vi "Initialize by XML.vi"(7 "XML File":path, 8 "error in (no error)":errorcluster, 10 "FPGA Device Address":string, 11 "FPGA Bitfile":path) -> (0 "error out":errorcluster, 3 "1553 Board out":refnum<class "1553 Board.lvclass">)   [LabVIEW 2016]
doc: "Generates a complete 1553 Board configuration when supplied a properly-formatted XML definition file.\n\nThe FPGA Bitfile must be one of the supported bitfiles that facilitates data communication with the 1553 Board. The FPGA Device Address must be a valid FPGA target."
uses:
  1553 Board.lvclass
  1553 Component/1553 Component.lvclass
  <vilib>/xml/NI_XML.lvlib
  <vilib>/xml/Load XML File.vi
  <vilib>/xml/Close Reference(Node).vi
  Utilities/FPGA Interface/FPGA Interface.lvclass
  Bus Controller/Bus Controller.lvclass
  D:/SVN/Products/BCI-1553/Software/Development/2016/Windows/1553 SubComponent/1553 SubComponent.lvclass
  Bus Monitor/Bus Monitor.lvclass
  Remote Terminal/Remote Terminal.lvclass
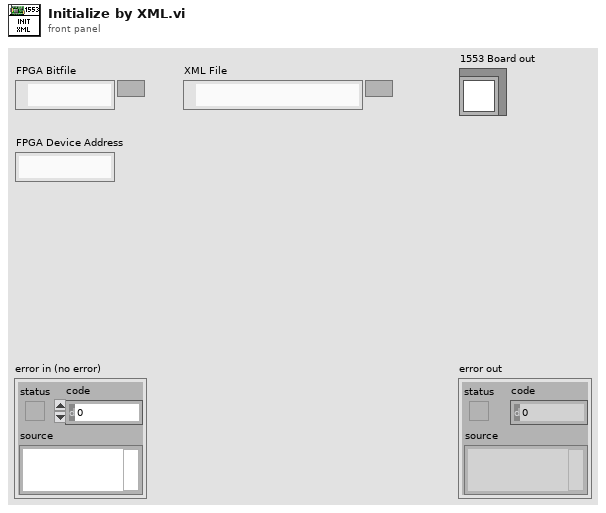
[diagram p1: front panel]
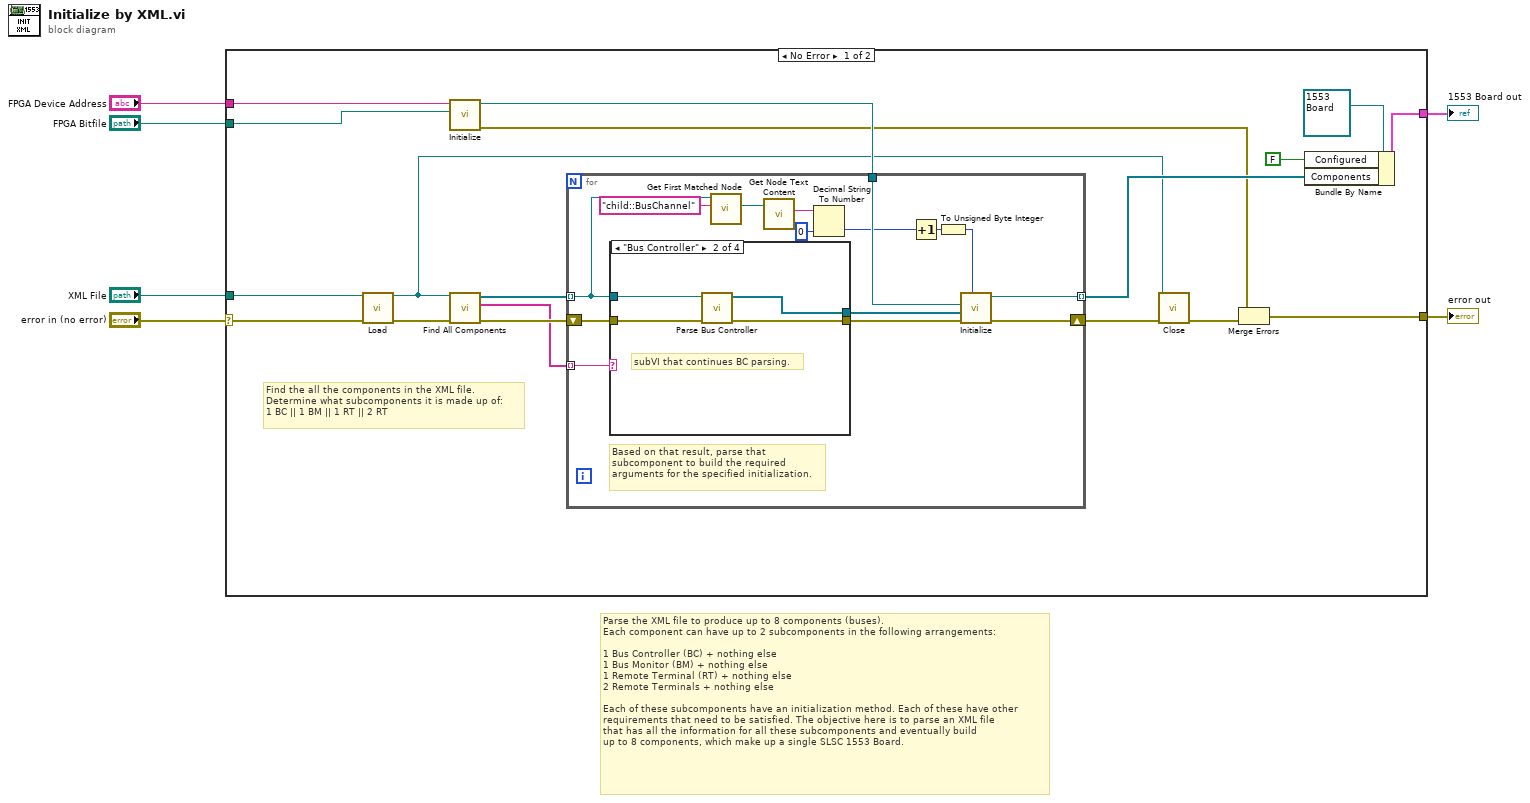
[diagram p0: block diagram]
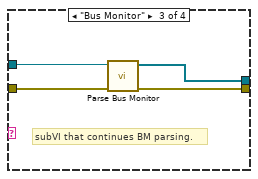
[diagram p3: hidden frame]
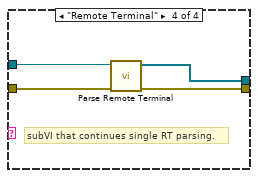
[diagram p4: hidden frame]
diagram:
  # "Parse the XML file to produce up to 8 components (buses).\nEach component can have up to 2 subcomponents in the following arrangements:\n\n1 Bus Controller (BC) + nothing else\n1 Bus Monitor (BM) + nothing else\n1 Remote Terminal (RT) + nothing else\n2 Remote Terminals + nothing else\n\nEach of these subcomponents have an initialization method. Each of these have other\nrequirements that need to be satisfied. The objective here is to parse an XML file\nthat has all the information for all these subcomponents and eventually build\nup to 8 components, which make up a single SLSC 1553 Board."
  n1 = case shown="No Error" "error in (no error)" {
    selector: "error in (no error)" -> [w16 w53]
    tunnel: [w7 w53] -> w5
    tunnel: [w23 _] -> w4
    tunnel: "FPGA Bitfile" -> [w21 _]
    tunnel: "FPGA Device Address" -> [w20 _]
    tunnel: "XML File" -> [w17 _]
    frame No Error {
      # "Find the all the components in the XML file.\nDetermine what subcomponents it is made up of:\n1 BC || 1 BM || 1 RT || 2 RT"
      n2 = call-poly <vilib>:"Load.vi"("path to XML document"=w17, "error in (no error)"=w16) -> ("DOM document out"=w14:refnum<k20>, "error out"=w13:errorcluster)  [unwired: 11 in, 1 out]
      n3 = call "Initialize.vi"("Bitfile path"=w21, "Device address"=w20) -> ("error out"=w9:errorcluster, "FPGA Interface out"=w19:refnum<class "FPGA Interface.lvclass">)  [unwired: 8 in]
      n4 = call "Find All Components.vi"("error in (no error)"=w13, "XML Doc Ref in"=w14) -> ("error out"=w12:errorcluster, "Component Types"=w10:string[], "Nodes"=w11:refnum<k20>[])  [unwired: 7 in]
      n5 = for {
        tunnel: w19 -> [w39]
        tunnel: [w31] -> w18 mode=indexing
        tunnel: w10 -> [w34] mode=indexing
        shift-right: [w38] -> w15
        shift-left: w12 -> [w33]
        tunnel: w11 -> [w30] mode=indexing
        # "Based on that result, parse that\nsubcomponent to build the required\narguments for the specified initialization."
        n6 = case shown="\"Bus Controller\"" w34 {
          tunnel: [w40 w42 w46 w50] -> w36
          tunnel: w33 -> [w40 w43 w48 w51]
          tunnel: [_ w41 w45 w49] -> w35
          tunnel: w30 -> [_ w44 w47 w52]
          frame Default {
            # "This case makes no sense.\nMake sure it doesn't get called."
          }
          frame "Bus Controller" {
            # "subVI that continues BC parsing."
            n7 = call "Parse Bus Controller.vi"("error in (no error)"=w43, "Bus Controller XML Node"=w44) -> ("error out"=w42:errorcluster, "Bus Controller"=w41:refnum<class "Bus Controller.lvclass">[])  [unwired: 8 in]
          }
          frame "Bus Monitor" {
            # "subVI that continues BM parsing."
            n8 = call "Parse Bus Monitor.vi"("error in (no error)"=w48, "Bus Monitor XML Node"=w47) -> ("error out"=w46:errorcluster, "Bus Monitor"=w45:refnum<class "Bus Monitor.lvclass">[])  [unwired: 8 in]
          }
          frame "Remote Terminal" {
            # "subVI that continues single RT parsing."
            n9 = call "Parse Remote Terminal.vi"("error in (no error)"=w51, "Single RT XML Node"=w52) -> ("error out"=w50:errorcluster, "Single RT"=w49:refnum<class "Remote Terminal.lvclass">[])  [unwired: 8 in]
          }
        }
        n10 = call <vilib>:"Get First Matched Node.vi"("XPath expression"="child::BusChannel", "node in"=w30) -> ("node result"=w28:refnum<k20>)  [unwired: 7 in, 2 out]
        n11 = call <vilib>:"Get Node Text Content.vi"("node in"=w28) -> ("node text"=w27:string)  [unwired: 8 in, 2 out]
        n12 = Decimal String To Number(string=w27, default (0L)=0 ("default (0 I32)")) -> (number=w25:i32)  [unwired: 1 in, 1 out]
        n13 = Increment(x=w25) -> (x+1=w37:i32)
        n14 = To Unsigned Byte Integer(number=w37) -> (unsigned 8bit integer=w32:u8)
        n15 = call "Initialize.vi"("Component ID (1-8)"=w32, "error in (no error)"=w36, "SubComponents"=w35, "FPGA Interface"=w39) -> ("error out"=w38:errorcluster, "1553 Component out"=w31:refnum<class "1553 Component.lvclass">)  [unwired: 6 in]
      }
      n16 = call-poly <vilib>:"Close.vi"("error in (no error)"=w15, "node"=w14) -> ("error out"=w8:errorcluster)  [unwired: 7 in]
      n17 = Merge Errors(w9, w8) -> (w7:errorcluster)
      n18 = Bundle By Name(cluster=refnum<class "1553 Board.lvclass"> refnum ("1553 Board out"), "Configured"=FALSE, "Components"=w18) -> (w23:cluster{})
    }
    frame Error {
    }
  }
  "error out" <- w5
  "1553 Board out" <- w4
